vi "Read Sweep configuration.vi"(8 "error in (no error)":errorcluster, 11 "Sweeper  in":refnum<class "Sweeper.lvclass">) -> (0 "error out":errorcluster, 2 "Sweep configuration":T1={"Set point"=0.0, "Sweep rate"=0.0, "Sweep action"=enum."To set point"}, 3 "Sweeper  out":refnum<class "Sweeper.lvclass">)   [LabVIEW 2018, in "Sweeper.lvclass"]
uses:
  Sweeper.lvclass
  C:/github/LabActor/Template Module/Template Module.lvclass
  NHMFL_Core/Libraries/Instruments/Controls/Set Output.ctl
  NHMFL_Core/Libraries/Instruments/Controls/Sweep Action.ctl
  Template Module/Template Module.lvclass/Template Module.ctl
  Template Module/Read Configuration.vi
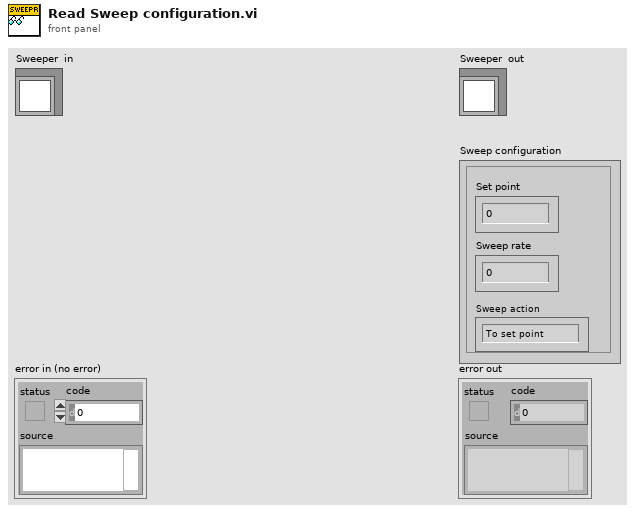
[diagram p1: front panel]
types:
  T1 = typedef "Set Output.ctl" = cluster{"Set point":dbl, "Sweep rate":dbl, "Sweep action":T2}
  T2 = typedef "Sweep Action.ctl" = enum16{"Hold", "To set point", "To zero", "Clamp"}
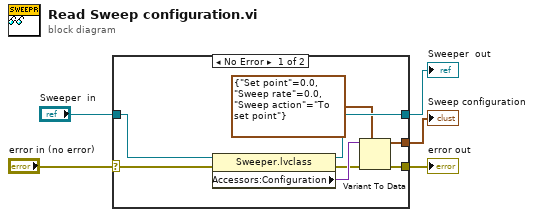
[diagram p0: block diagram]
diagram:
  n1 = case shown="No Error" "error in (no error)" {
    selector: "error in (no error)" -> [w7 w14]
    tunnel: [w11 w14] -> w4
    tunnel: [w12 w15] -> w2
    tunnel: "Sweeper  in" -> [w13 w15]
    tunnel: [w8 _] -> w1
    frame No Error {
      n2 = property class="Sweeper.lvclass"(reference=w13, error in=w7) -> (reference out=w12:refnum<class "Sweeper.lvclass">, error out=w6:errorcluster, "Accessors:Configuration"=w9:variant)
      n3 = Variant To Data(error in=w6, type=T1 {"Set point"=0.0, "Sweep rate"=0.0, "Sweep action"=enum."To set point"} ("Set output"), Variant=w9) -> (data=w8:T1, error out=w11:errorcluster)
    }
    frame Error {
    }
  }
  "error out" <- w4
  "Sweeper  out" <- w2
  "Sweep configuration" <- w1
